vi "temp_hygro_main.vi"(8 "error in":errorcluster) -> (0 "error out":errorcluster, 2 "Temperatur":dbl, 3 "luftfeuchtigkeit":dbl)   [LabVIEW 2013, in "TempHygro.lvlib"]
uses:
  lib/TempHygro.lvlib
panel:
  out "stop":bool=TRUE
  out "String":string
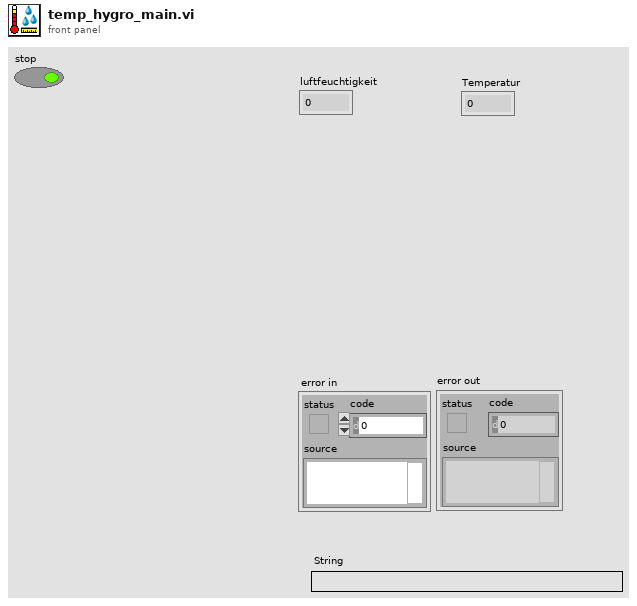
[diagram p1: front panel]
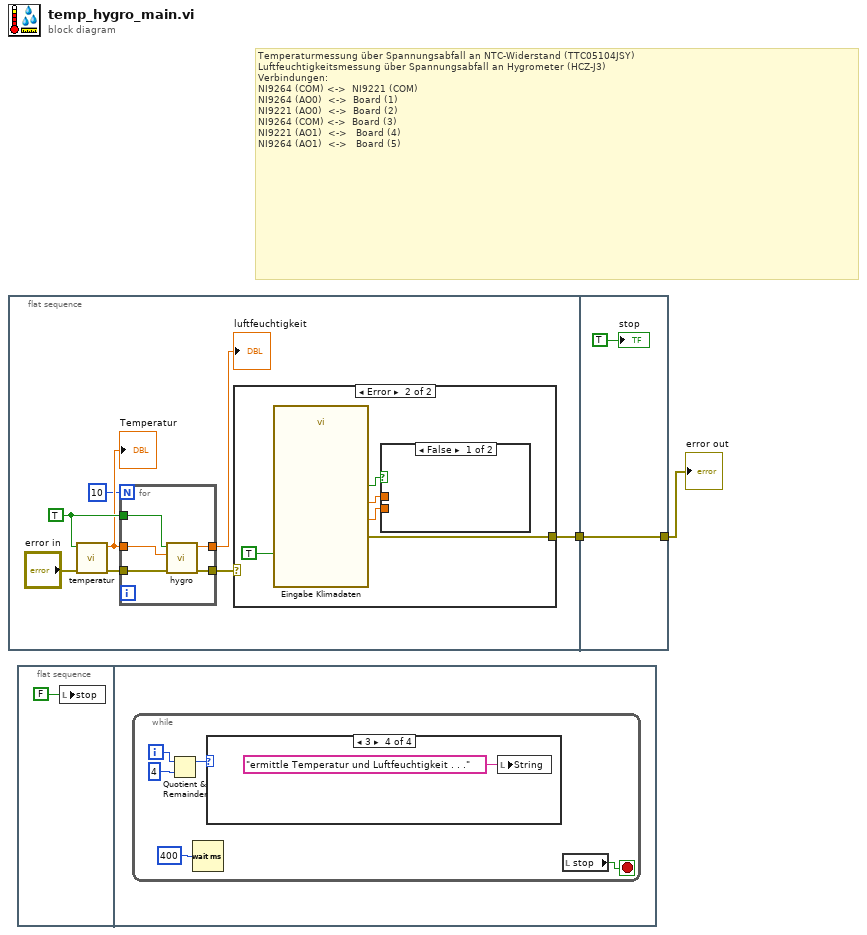
[diagram p0: block diagram]
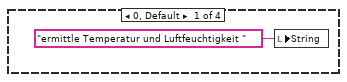
[diagram p2: hidden frame]
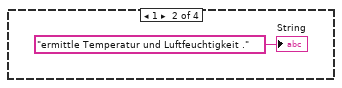
[diagram p3: hidden frame]
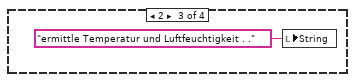
[diagram p4: hidden frame]
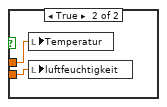
[diagram p6: hidden frame]
diagram:
  # "Temperaturmessung über Spannungsabfall an NTC-Widerstand (TTC05104JSY)\nLuftfeuchtigkeitsmessung über Spannungsabfall an Hygrometer (HCZ-J3)\nVerbindungen:  \nNI9264 (COM) <->  NI9221 (COM)\nNI9264 (AO0)  <->  Board (1)\nNI9221 (AO0)  <->  Board (2)\nNI9264 (COM) <->  Board (3)\nNI9221 (AO1)  <->   Board (4)\nNI9264 (AO1)  <->   Board (5)"
  n1 = flat-sequence {
    tunnel: [w3] -> w1
    tunnel: [w25] -> w2
    tunnel: w1 -> [w25]
    frame #0 {
      w9 = TRUE ("Start")
      n2 = call "temperatur.vi"("error in"="error in", "Start"=w9) -> ("error out"=w6:errorcluster, "Temperatur"=w7:dbl)  [unwired: 7 in, 1 out]
      "Temperatur" <- w7
      n3 = for {
        N: 10 -> [_]
        tunnel: [w23] -> w4
        tunnel: w9 -> [w22]
        tunnel: [w21] -> w8
        tunnel: w7 -> [w20]
        tunnel: w6 -> [w19]
        n4 = call "hygro.vi"("start"=w22, "temperatur"=w20, "Fehlerkonstante"=w19) -> ("luftfeuchtigkeit"=w21:dbl, "Fehlerkonstante 2"=w23:errorcluster)  [unwired: 4 in, 1 out]
      }
      "luftfeuchtigkeit" <- w8
      n5 = case shown="Error" w4 {
        selector: w4 -> [w11 _]
        tunnel: [w11 w16] -> w3
        frame No Error {
        }
        frame Error {
          n6 = call "Eingabe Klimadaten"("Enable"=TRUE) -> ("Luftfeuchtigkeit"=w14:dbl, "Temperatur"=w15:dbl, "OK"=w13:bool, "error out"=w16:errorcluster)  [unwired: 15 in]
          n7 = case shown="False" w13 {
            tunnel: w15 -> [_ w18]
            tunnel: w14 -> [_ w17]
            frame False {
            }
            frame True {
              n8 = local write "Temperatur"(w18) -> ()
              n9 = local write "luftfeuchtigkeit"(w17) -> ()
            }
          }
        }
      }
    }
    frame #1 {
      "stop" <- TRUE ("stop")
    }
  }
  n10 = flat-sequence {
    frame #0 {
      n11 = local write "stop"(FALSE ("stop")) -> ()
    }
    frame #1 {
      n12 = while {
        i -> [w30]
        stop <- w27 stop-if-true
        n13 = Quotient & Remainder(x=w30, y=4) -> (x-y*floor(x/y)=w28:i32)  [unwired: 1 out]
        n14 = Wait (ms)(milliseconds to wait=u32 400) -> ()  [unwired: 1 out]
        n15 = case shown="3" w28 {
          frame 0, Default {
            n16 = local write "String"("ermittle Temperatur und Luftfeuchtigkeit " ("String")) -> ()
          }
          frame 1 {
            "String" <- "ermittle Temperatur und Luftfeuchtigkeit ." ("String")
          }
          frame 2 {
            n17 = local write "String"("ermittle Temperatur und Luftfeuchtigkeit . ." ("String")) -> ()
          }
          frame 3 {
            n18 = local write "String"("ermittle Temperatur und Luftfeuchtigkeit . . ." ("String")) -> ()
          }
        }
        n19 = local read "stop"() -> (w27:bool)
      }
    }
  }
  "error out" <- w2
